vi "Configure Protect Curr.vi"(8 "error in (no error)":errorcluster, 9 "Curr(0)":dbl min=0.0 max=300.0, 10 "Enable":bool, 11 "VISA resource name":refnum<visa-resource-name>) -> (0 "error out":errorcluster, 3 "VISA resource name out":refnum<visa-resource-name>)   [LabVIEW 2020, in "IT6500.lvlib"]
doc: "This command opens or closes the current protection function.And it is used to set the upper limit of current protection OCP."
uses:
  IT6500.lvlib
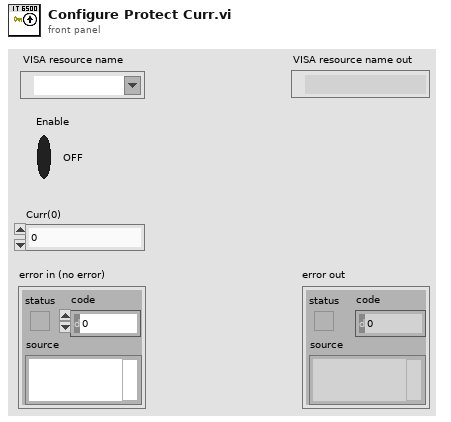
[diagram p1: front panel]
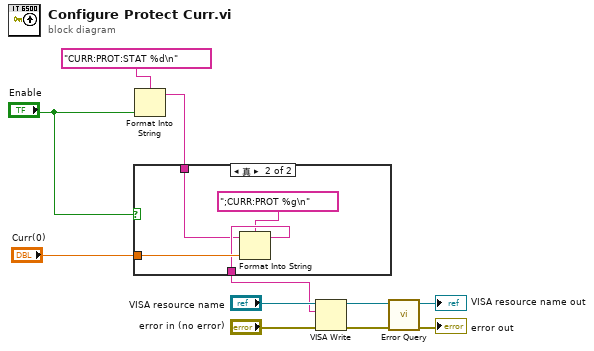
[diagram p0: block diagram]
diagram:
  n1 = Format Into String(format string="CURR:PROT:STAT %d\n", "Enable") -> (resulting string=w4:string)  [unwired: 2 in, 1 out]
  n2 = case shown="真" "Enable" {
    tunnel: w4 -> [w12 w13]
    tunnel: "Curr(0)" -> [_ w16]
    tunnel: [w12 w15] -> w1
    frame False {
    }
    frame True {
      n3 = Format Into String(format string=";CURR:PROT %g\n", initial string=w13, w16) -> (resulting string=w15:string)  [unwired: 1 in, 1 out]
    }
  }
  n4 = VISA Write(VISA resource name="VISA resource name", write buffer=w1, error in (no error)="error in (no error)") -> (VISA resource name out=w8:refnum<visa-resource-name>, error out=w9:errorcluster)  [unwired: 1 out]
  n5 = call "Error Query.vi"("error in (no error)"=w9, "VISA resource name"=w8) -> ("error out"=→"error out":errorcluster, "VISA resource name out"=→"VISA resource name out":refnum<visa-resource-name>)  [unwired: 6 in, 2 out]
